vi "RRTPlan.vi"(8 "Initial Pos x,y":dbl[](array[numeric]), 9 "Dest x,y":dbl[](array[numeric]), 10 "IA State":T3={"our_robots"=[], "enemy_robots"=[], "balls"=[], "geometry"={"field_length"=0, "field_width"=0, "goal_width"=0, "goal_depth"=0, "center_circle_radius"=0, "defense_width"=0, "defense_depth"=0, "free_kick_from_defense_dist"=0, "penalty_spot_from_field_line_dist"=0, "penalty_line_from_spot_dist"=0, "half_moon_depth"=0, "half_moon_width"=0}, "IA Judge"={"stage"="", "command"="", "our_goalie_id"=0.0, "enemy_goalie_id"=0.0, "command enum"=enum."Halt", "Time"=enum."Azul"}, "Received Timestamp"=timestamp(0 s since 1904-01-01), "Events"={"Touch"=FALSE, "Ball out"=FALSE, "id touch"=0.0, "Ball out of \nVision"=FALSE, "Ball inside \nGoalie area"=FALSE, "Robot not responding"=FALSE, "Robots responding status"=[1.0, 1.0, 1.0, 1.0, 1.0, 1.0], "Enemy Ball \nPossession"=FALSE, "Pass State"=FALSE, "id end of pass"=0.0, "Kick"=FALSE, "Id ini Possession"=0.0, "Ball Possesion"=FALSE, "Id Possesion"=0.0}}, 11 "Robot":T4={"id"=0, "function"=enum."Attacker", "x"=0.0, "y"=0.0, "orientation"=0.0, "v_tangent"=0.0, "v_normal"=0.0, "v_ang"=0.0, "kick_x"=0.0, "kick_z"=0.0, "dribble"=FALSE, "Timestamp"=timestamp(0 s since 1904-01-01), "estimatives"={"est_v_tangent"=0.0, "est_v_normal"=0.0, "est_vx"=0.0, "est_vy"=0.0, "Pos Robot Est"=[]}, "dest_x_kick"=0.0, "dest_y_kick"=0.0, "Gap Coord"=[], "States"=enum."GoToTangent", "Path "=[], "Path  Smooth"=[], "Dest"=[]}) -> (0 "Path":dbl[][](array[numeric]), 1 "Smooth Path":dbl[][](array[numeric]))   [LabVIEW 2017]
uses:
  Core/AI Robot.ctl
  Intel/Functions Enum.ctl
  Intel/AttackerStates.ctl
  PathDests.ctl
  PathDest.ctl
  Core/AI Input.ctl
  Core/AI Ball.ctl
  Core/Field Size.ctl
  Core/AI Judge.ctl
  Intel/Command Enum.ctl
  Util/Events/Events.ctl
  kD-tree/KD-Tree.ctl
  kD-tree/Node.ctl
  <vilib>/Analysis/_algsub.llb/Real Vector Norm.vi
  <vilib>/Analysis/NI_AALPro.lvlib
panel:
  out "New KD-Tree":T1
  out "x > y? 2":bool
  out "Modulo":dbl
  in  "WayPointProb":dbl=0.6 format="%#_13g"
  in  "GoalProb":dbl=0.1 format="%#_13g"
  in  "Step":dbl=80.0
  out "Elapsed Time (s)":dbl
  out "Time has Elapsed":bool
  in  "threshold":dbl=80.0
  out "Goal":dbl[](array[numeric])
  out "Initial State":dbl[](array[numeric])
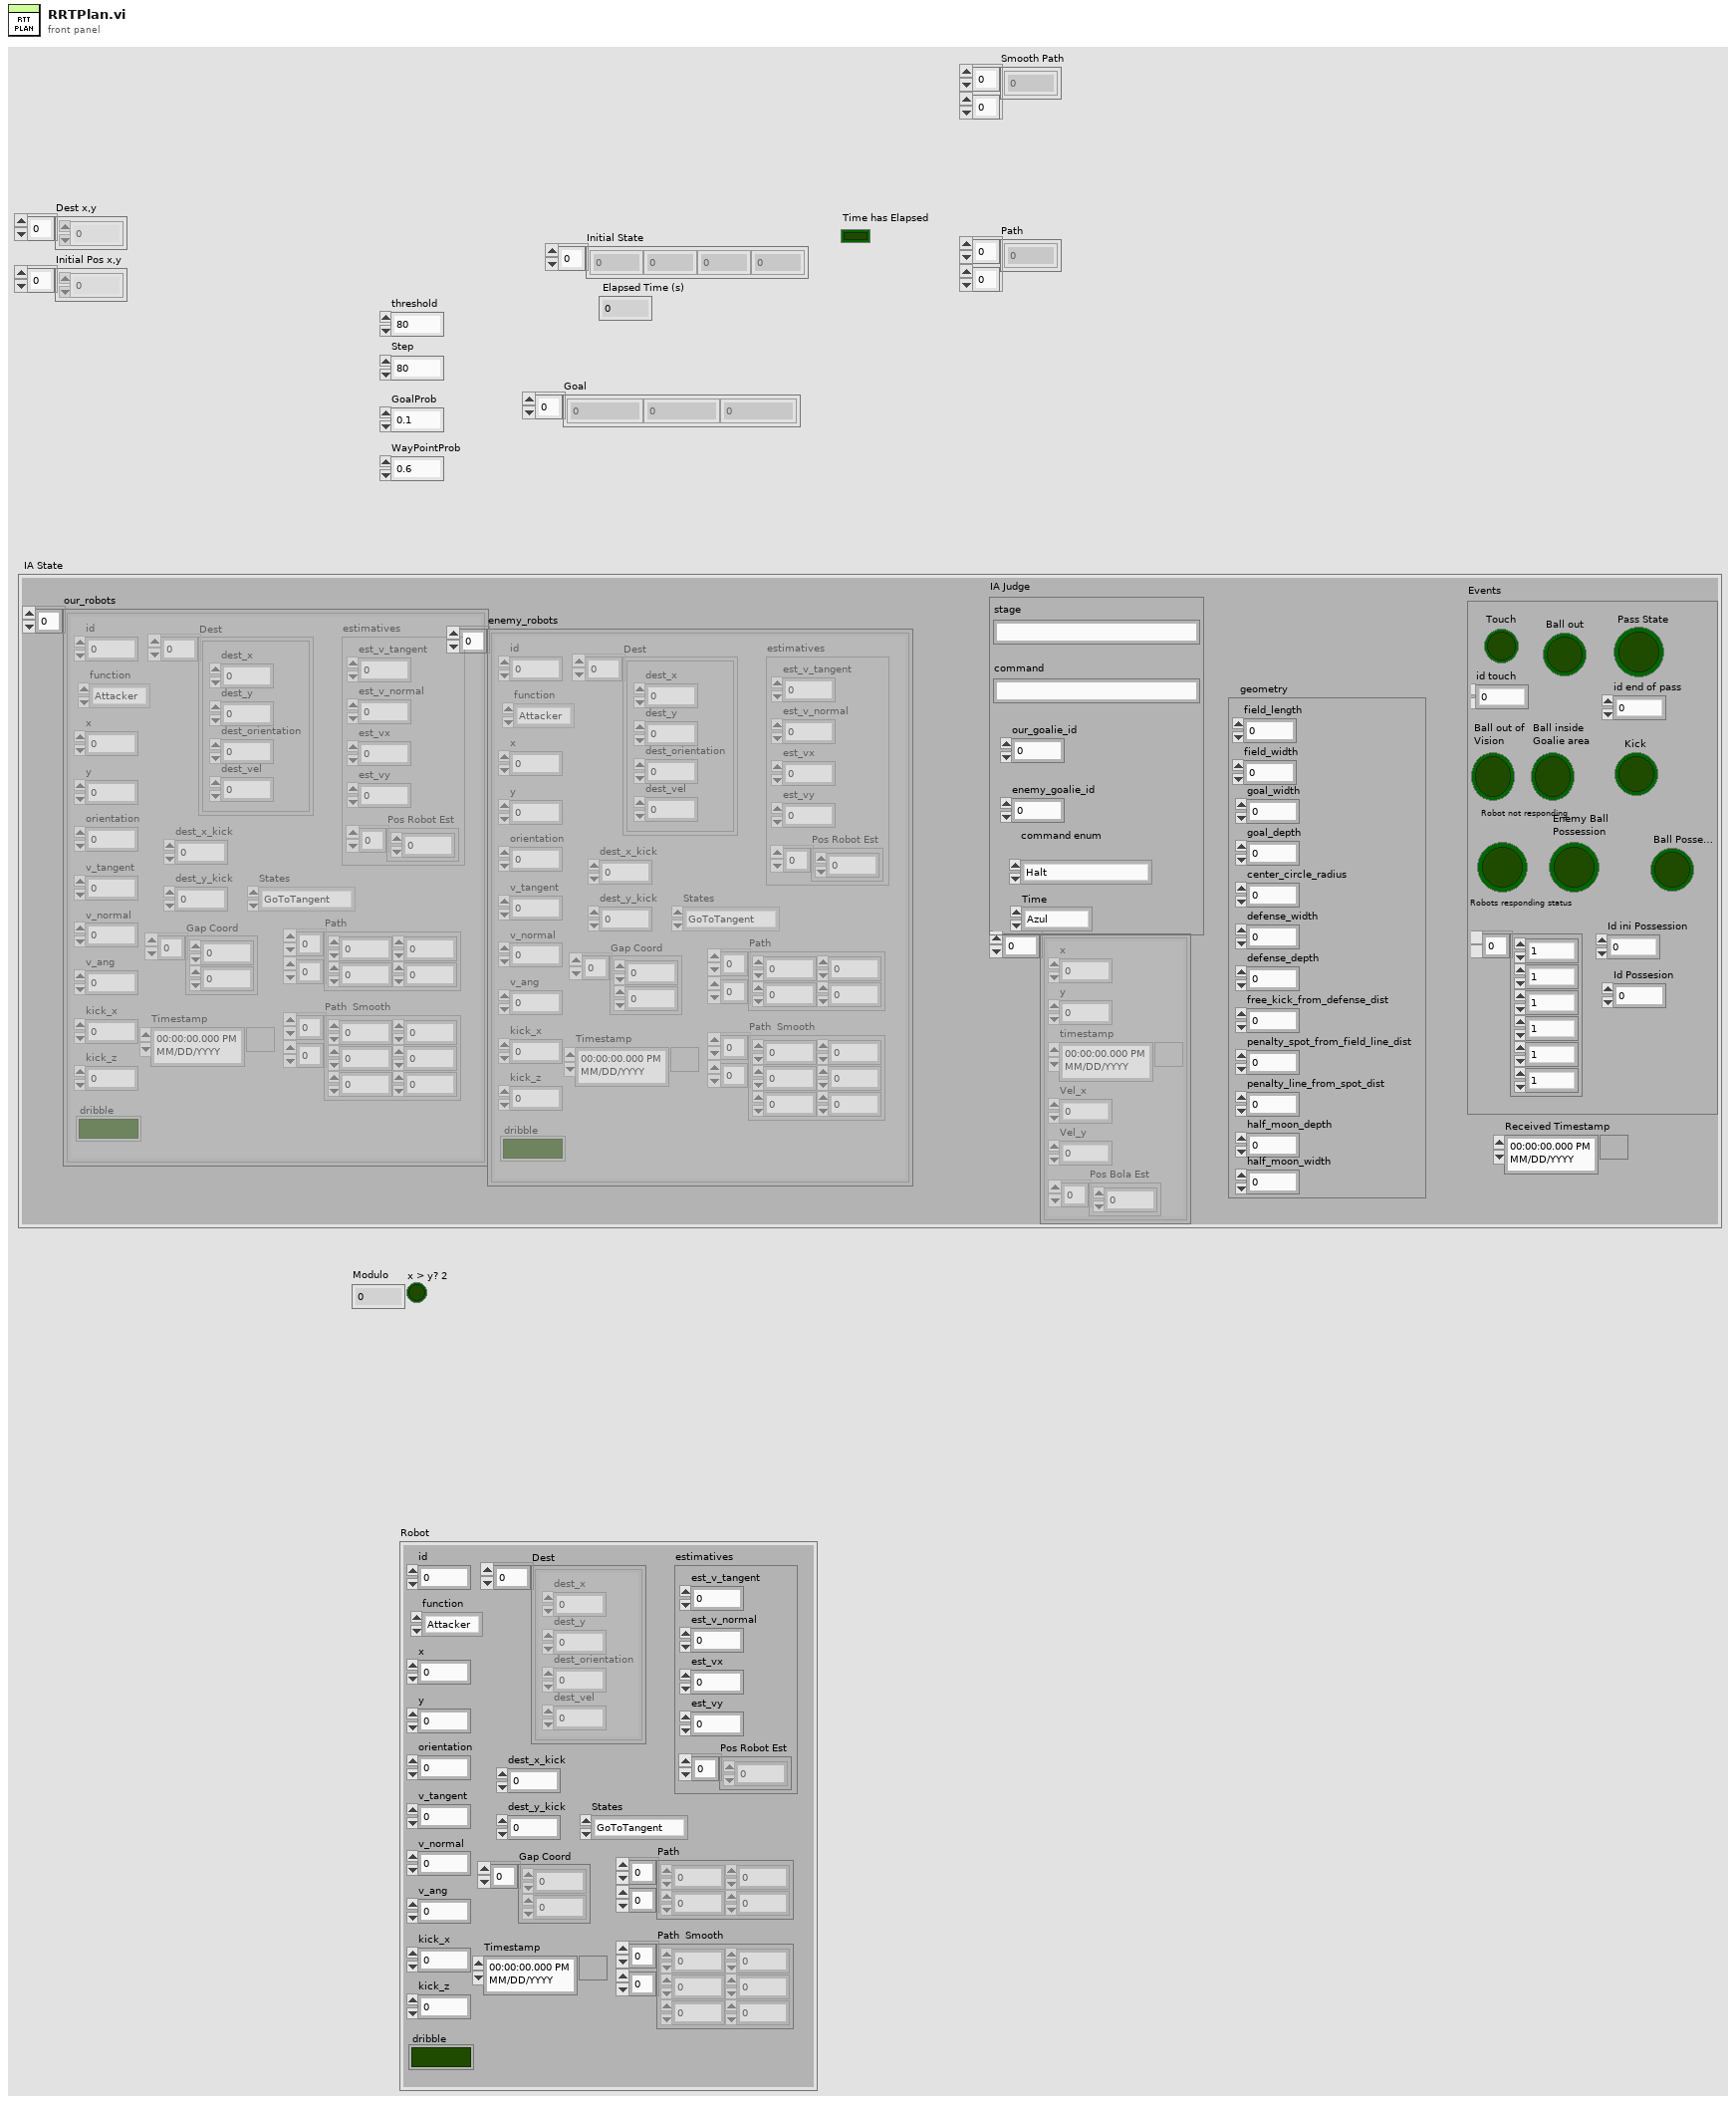
[diagram p1: front panel]
types:
  T1 = typedef "KD-Tree.ctl" = T2[]
  T2 = typedef "Node.ctl" = cluster{"axis":enum16{"null", "x", "y"}, "value":dbl, "left":dbl, "right":dbl, "Point":dbl[]}
  T3 = typedef "AI Input.ctl" = cluster{"our_robots":T4[], "enemy_robots":T4[], "balls":T9[], "geometry":T10, "IA Judge":T11, "Received Timestamp":timestamp, "Events":T13}
  T4 = typedef "AI Robot.ctl" = cluster{"id":u32, "function":T5, "x":dbl, "y":dbl, "orientation":dbl, "v_tangent":dbl, "v_normal":dbl, "v_ang":dbl, "kick_x":dbl, "kick_z":dbl, "dribble":bool, "Timestamp":timestamp, "estimatives":cluster{"est_v_tangent":dbl, "est_v_normal":dbl, "est_vx":dbl, "est_vy":dbl, "Pos Robot Est":dbl[]}, "dest_x_kick":dbl, "dest_y_kick":dbl, "Gap Coord":dbl[], "States":T6, "Path ":dbl[][], "Path  Smooth":dbl[][], "Dest":T7}
  T5 = typedef "Functions Enum.ctl" = enum16{"Attacker", "Goalie", "Defender", "Striker", "Goto 0", "Dummy", "Kicker", "ZigZag"}
  T6 = typedef "AttackerStates.ctl" = enum16{"Pass", "GoToTangent", "BallGetting", "GoToKick", ""}
  T7 = typedef "PathDests.ctl" = T8[]
  T8 = typedef "PathDest.ctl" = cluster{"dest_x":dbl, "dest_y":dbl, "dest_orientation":dbl, "dest_vel":dbl}
  T9 = typedef "AI Ball.ctl" = cluster{"x":dbl, "y":dbl, "timestamp":timestamp, "Vel_x":dbl, "Vel_y":dbl, "Pos Bola Est":dbl[]}
  T10 = typedef "Field Size.ctl" = cluster{"field_length":u32, "field_width":u32, "goal_width":u32, "goal_depth":u32, "center_circle_radius":u32, "defense_width":u32, "defense_depth":u32, "free_kick_from_defense_dist":u32, "penalty_spot_from_field_line_dist":u32, "penalty_line_from_spot_dist":u32, "half_moon_depth":u32, "half_moon_width":u32}
  T11 = typedef "AI Judge.ctl" = cluster{"stage":string, "command":string, "our_goalie_id":dbl, "enemy_goalie_id":dbl, "command enum":T12, "Time":enum16{"Azul", "Amarelo"}}
  T12 = typedef "Command Enum.ctl" = enum16{"Halt", "Stop", "Force Start", "PKA Normal Start", "Prepare Kickoff Ally", "PKE Normal Start", "Prepare Kickoff Enemy", "Prepare Penalty Ally", "PPA Normal Start", "Prepare Penalty Enemy", "PPE Normal Start", "Direct Free Enemy", "Direct Free Ally", "Indirect Free Enemy", "Indirect Free Ally", "Timeout Enemy", "Timeout Ally", "Goal Enemy", "Goal Ally", "Ball Placement Enemy", "Ball Placement Ally", "Normal Half Time", "Extra Time Break", "Extra Half Time", "None", "Post Game"}
  T13 = typedef "Events.ctl" = cluster{"Touch":bool, "Ball out":bool, "id touch":dbl, "Ball out of \nVision":bool, "Ball inside \nGoalie area":bool, "Robot not responding":bool, "Robots responding status":dbl[], "Enemy Ball \nPossession":bool, "Pass State":bool, "id end of pass":dbl, "Kick":bool, "Id ini Possession":dbl, "Ball Possesion":bool, "Id Possesion":dbl}
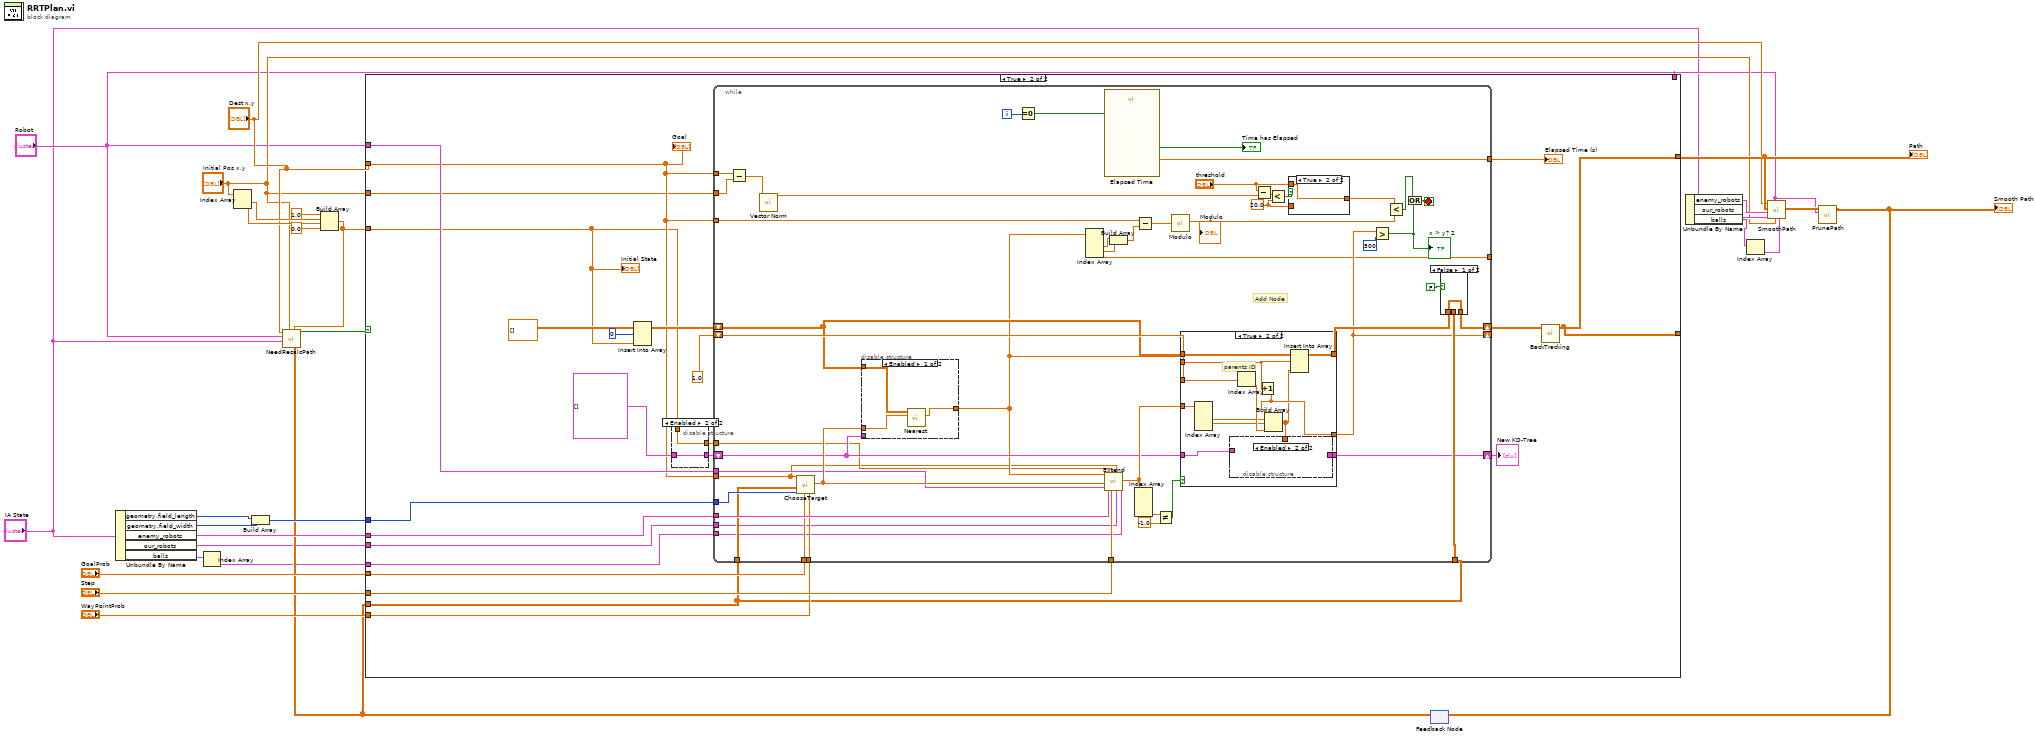
[diagram p0: block diagram]
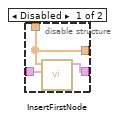
[diagram p3: hidden frame]
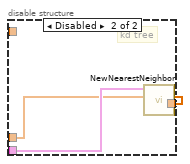
[diagram p4: hidden frame]
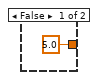
[diagram p5: hidden frame]
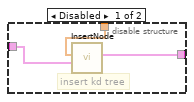
[diagram p8: hidden frame]
diagram:
  n1 = Unbundle By Name("IA State") -> ("geometry.field_length"=w28:u32, "geometry.field_width"=w27:u32, "enemy_robots"=w22:T4[], "our_robots"=w17:T4[], "balls"=w2:T9[])
  n2 = Index Array(array=w2) -> (element=w1:T9)  [unwired: 1 in]
  n3 = Index Array(array="Initial Pos x,y") -> (element #1=w16:dbl, element #2=w15:dbl)  [unwired: 2 in]
  n4 = Build Array(w28, w27) -> (w26:u32[])
  n5 = Build Array(1.0 ("element"), w16, w15, 0.0 ("element")) -> (w19:dbl[])
  n6 = feedback #1() -> (w18:dbl[][])  [unwired: 1 in]
  n7 = call "NeedRecalcPath.vi"("SmoothPath"=w18, "Initial State"=w19, "Pos x,y"="Initial Pos x,y", "IA State"="IA State", "Robot"="Robot", "Dest x,y"="Dest x,y") -> ("Boolean"=w5:bool)  [unwired: 5 in]
  n8 = case shown="True" w5 {
    tunnel: w26 -> [_ w42]
    tunnel: "Step" -> [_ w49]
    tunnel: "Robot" -> [_ w37]
    tunnel: "GoalProb" -> [_ w47]
    tunnel: "WayPointProb" -> [_ w46]
    tunnel: w22 -> [_ w45]
    tunnel: w18 -> [w29 w44]
    tunnel: [w29 w35] -> w12
    tunnel: "Robot" -> [_ _]
    tunnel: [w29 w35] -> _
    tunnel: "Dest x,y" -> [_ w34]
    tunnel: "Initial Pos x,y" -> [_ w33]
    tunnel: w19 -> [_ w32]
    tunnel: w17 -> [_ w31]
    tunnel: w1 -> [_ w30]
    frame False {
    }
    frame True {
      n9 = Insert Into Array(array=dbl[][] [] ("Pontos"), index (row)=0, new element=w32) -> (w50:dbl[][])  [unwired: 1 in]
      n10 = disable-structure shown="Enabled" {
        disable-tunnel: [w55 w57] -> w40
        disable-tunnel: T1 [] ("New KD-Tree") -> [w54 w57]
        disable-tunnel: w32 -> [w53 w56]
        disable-tunnel: [w53 w56] -> w36
        frame Disabled {
          n11 = call "InsertFirstNode.vi"("New KD-Tree in"=w54, "Tree"=w53) -> ("New KD-Tree out"=w55:T1)  [unwired: 9 in]
        }
        frame Enabled {
        }
      }
      n12 = while {
        tunnel: w34 -> [w106]
        tunnel: w34 -> [w61]
        tunnel: w42 -> [w103]
        shift-right: [w87] -> w43
        shift-left: w50 -> [w86]
        tunnel: w45 -> [w101]
        tunnel: w49 -> [w100]
        shift-right: [w83] -> _
        shift-left: 1.0 -> [w91]
        tunnel: w44 -> [w90]
        tunnel: w44 -> [w89]
        tunnel: w47 -> [w81]
        tunnel: w46 -> [w80]
        tunnel: [w77] -> _
        tunnel: w34 -> [w76]
        shift-right: [w69] -> w41
        shift-left: w40 -> [w68]
        tunnel: [w66] -> w38
        tunnel: w37 -> [w63]
        tunnel: w36 -> [w62]
        tunnel: w33 -> [w60]
        tunnel: w31 -> [w59]
        tunnel: w30 -> [w58]
        i -> [w65]
        stop <- w95 stop-if-true
        w70 = 20.0 ("y")
        # "Add Node"
        n13 = Subtract(x=w76, y=w60) -> (x-y=w75:dbl[])
        n14 = call-poly <vilib>:"Vector Norm.vi"("Input Vector"=w75) -> ("norm"=w73:dbl)  [unwired: 9 in, 1 out]
        n15 = call "ChooseTarget.vi"("WayPointProb"=w80, "GoalProb"=w81, "Field Geometry"=w103, "WayPointCache"=w90, "Goal"=w61) -> ("Target"=w102:dbl[])  [unwired: 6 in]
        n16 = disable-structure shown="Enabled" {
          disable-tunnel: w102 -> [w110 w112]
          disable-tunnel: w86 -> [w109 _]
          disable-tunnel: w68 -> [_ w113]
          disable-tunnel: [w108 w111] -> w67
          frame Enabled {
            n17 = call "Nearest.vi"("Target"=w110, "Pontos"=w109) -> ("Nearest"=w108:dbl[])  [unwired: 9 in]
          }
          frame Disabled {
            # "kd tree"
            n18 = call "NewNearestNeighbor.vi"("q"=w112, "KD-Tree"=w113) -> ("Nearest"=w111:dbl[])  [unwired: 9 in]
          }
        }
        n19 = Equal To 0?(x=w65) -> (x = 0?=w64:bool)
        n20 = Index Array(array=w67) -> (element #2=w94:dbl, element #3=w93:dbl, element #4=w77:dbl)  [unwired: 4 in, 1 out]
        n21 = call "Elapsed Time"("Auto Reset"=w64) -> ("Elapsed Time (s)"=w66:dbl, "Time has Elapsed"=→"Time has Elapsed":bool)  [unwired: 11 in, 6 out]
        n22 = call "Extend.vi"("Ball"=w58, "our_robots"=w59, "Goal"=w61, "Step"=w100, "Initial State"=w62, "enemy_robots"=w101, "Robot in"=w63, "Target"=w102, "Nearest"=w67) -> ("New State"=w96:dbl[])  [unwired: 2 in]
        n23 = Build Array(w94, w93) -> (w92:dbl[])
        n24 = Index Array(array=w96) -> (element #4=w99:dbl)  [unwired: 4 in, 3 out]
        n25 = Subtract(x=w106, y=w92) -> (x-y=w107:dbl[])
        n26 = Not Equal?(x=w99, y=-1.0) -> (x != y?=w97:bool)
        n27 = call "Modulo.vi"("2D vector"=w107) -> ("Modulo"=w105:dbl)  [unwired: 10 in]
        "Modulo" <- w105
        n28 = case shown="True" w97 {
          tunnel: w86 -> [w120 w132]
          tunnel: [w120 w128] -> w88
          tunnel: w96 -> [_ w131]
          tunnel: w91 -> [w119 w127]
          tunnel: w67 -> [_ w130]
          tunnel: [w119 w122] -> w83
          tunnel: [w118 w126] -> w69
          tunnel: w68 -> [w118 w125]
          frame False {
          }
          frame True {
            # "parents ID"
            n29 = Index Array(array=w131) -> (element #2=w124:dbl, element #3=w123:dbl)  [unwired: 4 in, 2 out]
            n30 = Index Array(array=w130) -> (element=w129:dbl)  [unwired: 1 in]
            n31 = Increment(x=w127) -> (x+1=w122:dbl)
            n32 = Build Array(w122, w124, w123, w129) -> (w121:dbl[])
            n33 = disable-structure shown="Enabled" {
              disable-tunnel: [w135 _] -> w126
              disable-tunnel: w125 -> [w134 _]
              disable-tunnel: w121 -> [w133 _]
              frame Disabled {
                # "insert kd tree"
                n34 = call "InsertNode.vi"("KD-Tree"=w134, "New Node"=w133) -> ("New KD-Tree"=w135:T1)  [unwired: 9 in]
              }
              frame Enabled {
              }
            }
            n35 = Insert Into Array(array=w132, index (row)=w127, new element=w121) -> (w128:dbl[][])  [unwired: 1 in]
          }
        }
        n36 = Subtract(x="threshold", y=w73) -> (x-y=w71:dbl)
        n37 = Less?(x=w71, y=w70) -> (x < y?=w72:bool)
        n38 = case shown="True" w72 {
          tunnel: [5.0 ("threshold") w115] -> w104
          tunnel: "threshold" -> [_ w115]
          tunnel: w70 -> [_ _]
          frame False {
          }
          frame True {
          }
        }
        n39 = Greater?(x=w83, y=500) -> (0:w78:bool)
        "x > y? 2" <- w78
        n40 = Less?(x=w105, y=w104) -> (x < y?=w79:bool)
        n41 = Or(x=w79, y=w78) -> (x .or. y?=w95:bool)
        n42 = case shown="False" FALSE {
          tunnel: w89 -> [_ w117]
          tunnel: [w116 w117] -> w87
          tunnel: w88 -> [w116 _]
          frame False {
          }
          frame True {
          }
        }
      }
      "New KD-Tree" <- w41
      "Elapsed Time (s)" <- w38
      n43 = call "BackTracking.vi"("Pontos"=w43) -> ("Path"=w35:dbl[][])  [unwired: 9 in, 1 out]
      "Initial State" <- w32
      "Goal" <- w34
    }
  }
  "Path" <- w12
  n44 = Unbundle By Name("IA State") -> ("enemy_robots"=w13:T4[], "our_robots"=w14:T4[], "balls"=w4:T9[])
  n45 = Index Array(array=w4) -> (element=w3:T9)  [unwired: 1 in]
  n46 = call "SmoothPath.vi"("ball"=w3, "Initial State"="Initial Pos x,y", "Robot in"="Robot", "our_robots"=w14, "enemy_robots"=w13, "Path"=w12, "Goal"="Dest x,y") -> ("SmoothPath"=w9:dbl[][])  [unwired: 4 in]
  n47 = call "PrunePath.vi"("Robot in"="Robot", "Path in"=w9) -> ("Path out"=w8:dbl[][])  [unwired: 8 in, 1 out]
  "Smooth Path" <- w8
  n48 = feedback-in #1(w8) -> ()
